vi "main.vi"() -> ()   [LabVIEW 2025]
uses:
  Controls/States.ctl
  Controls/HR_Data_Structure.ctl
  Controls/Raw_Data_IN_HR.ctl
  Controls/Runner_Data_Structure.ctl
  <vilib>/Analysis/baseanly.llb/Mean (DBL).vi
  <vilib>/Analysis/NI_AALBase.lvlib
panel:
  out "BPM":cluster{"Time":timestamp[], "Bpm":i32[]}(graph)
  out "Zone PLOT":T1(graph)
  out "Zone Data":string[][](array[string]) caption="HEART RATE ZONES"
  in  "File Path":path
  out "error out":errorcluster
  in  "error in":errorcluster
  in  "Stop":bool
  in  "Save Results":bool
  in  "New Training":bool
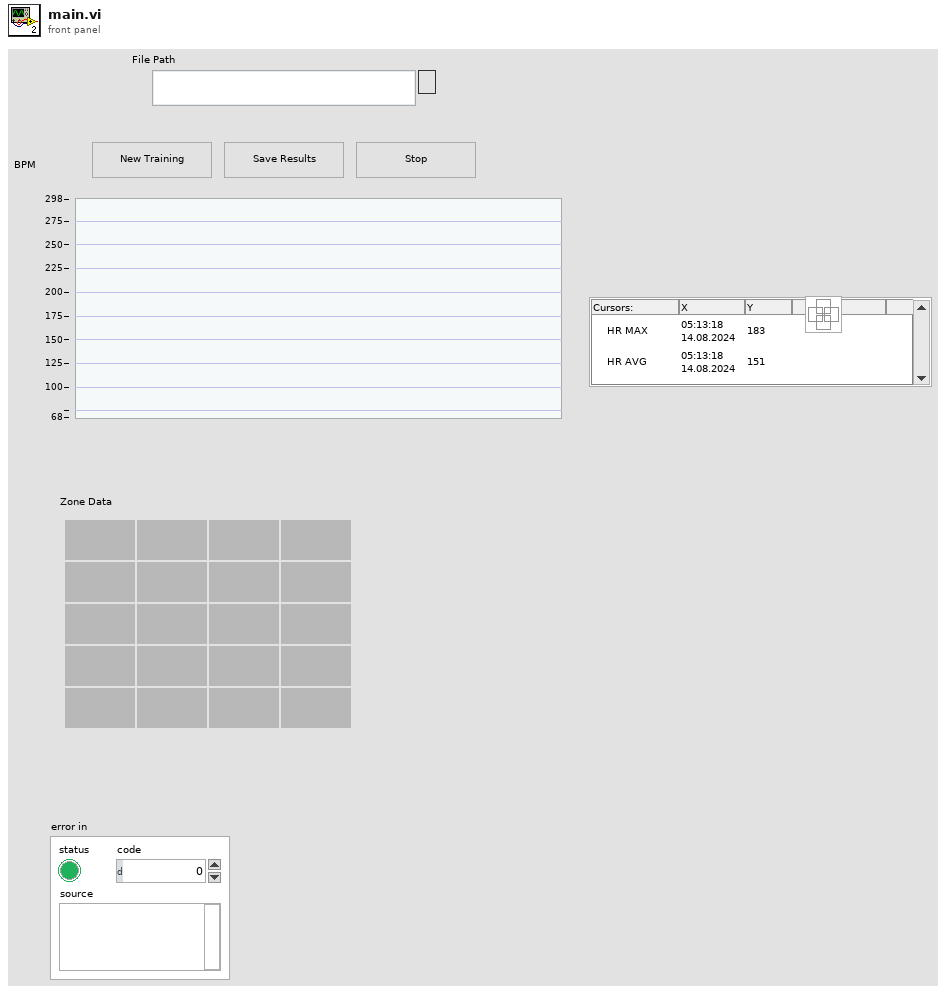
[diagram p1: front panel]
types:
  T1 = cluster{"Total Time in Zone":dbl[], "Heart Rate Zone No":dbl[]}
  T2 = typedef "HR_Data_Structure.ctl" = cluster{"HR Max":i32, "% HR MAX ":dbl[], "Raw Data":T3, "Runner's Data":T4, "HR Zone":string[][], "Total Time in Zone":dbl[], "Heart Rate Zone No":dbl[]}
  T3 = typedef "Raw_Data_IN_HR.ctl" = cluster{"Time":timestamp[], "Bpm":i32[]}
  T4 = typedef "Runner_Data_Structure.ctl" = cluster{"Name":string, "Age":i32}
  T5 = typedef "States.ctl" = enum16{"Application Error", "Init", "Idle", "Analyse New Training", "Save", "Error Handling", "Stop"}
  T6 = enum16{"open", "replace", "create", "open or create", "replace or create", "replace or create with confirmation"}
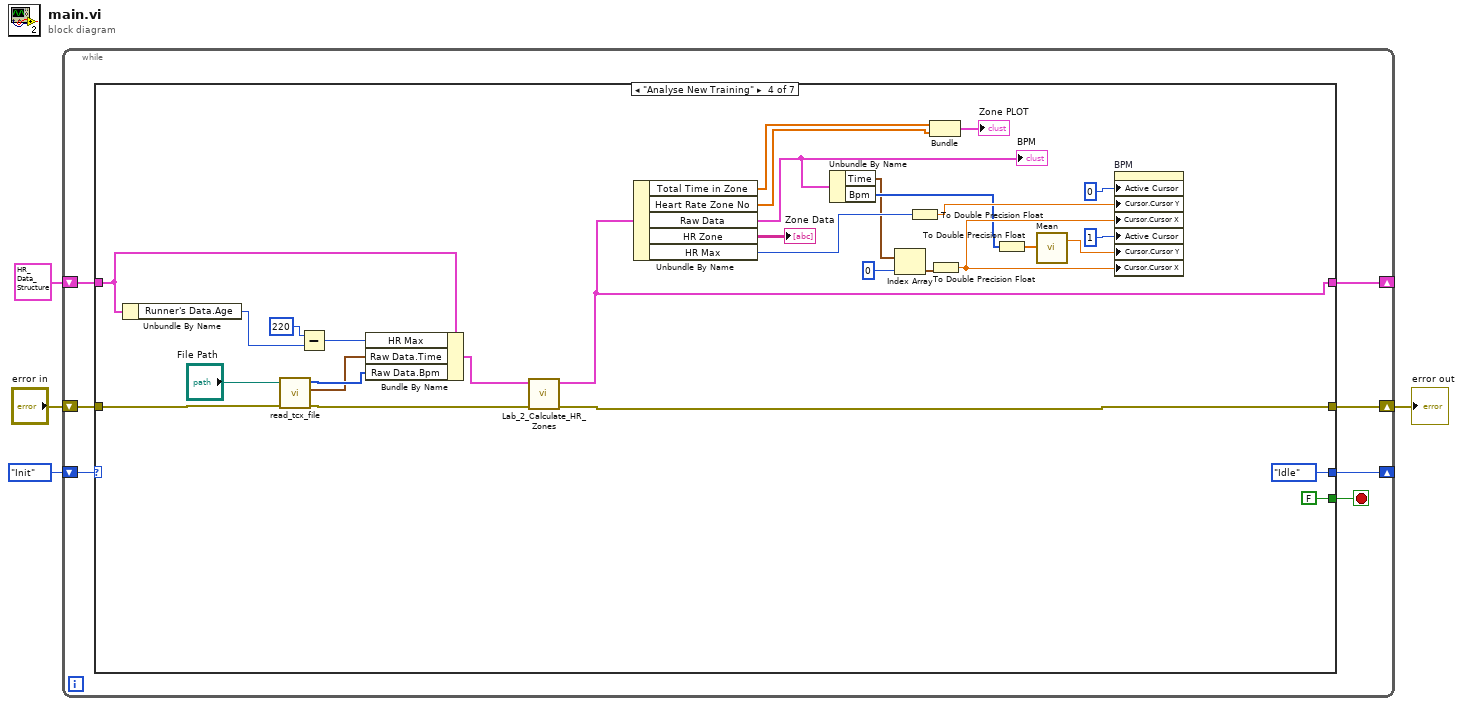
[diagram p0: block diagram]
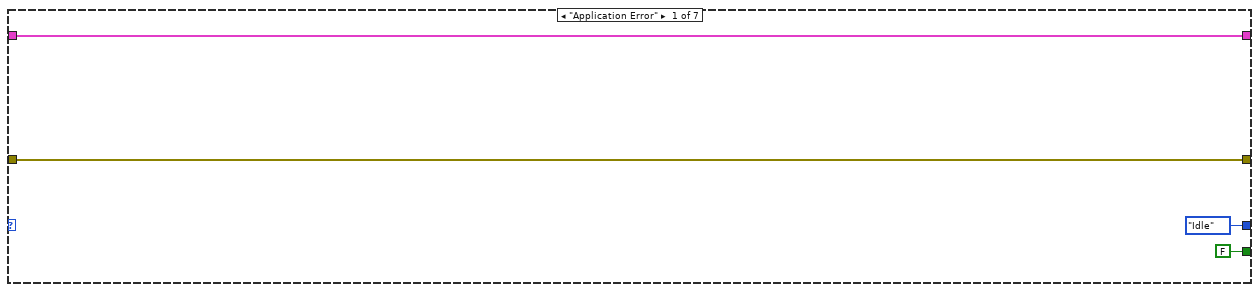
[diagram p2: hidden frame]
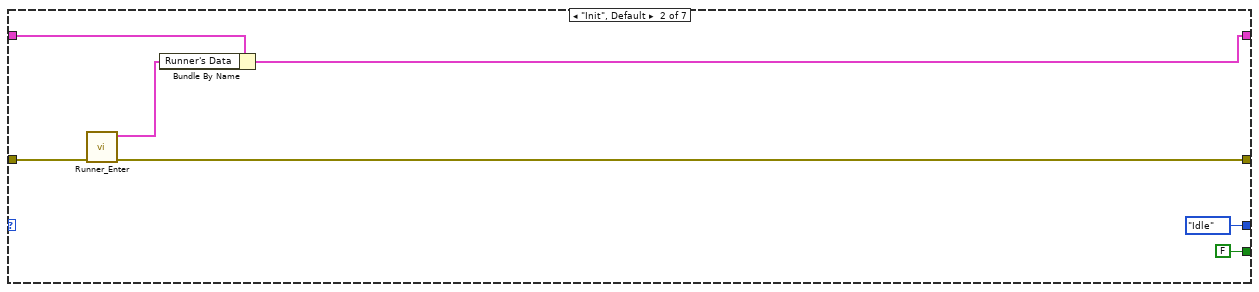
[diagram p3: hidden frame]
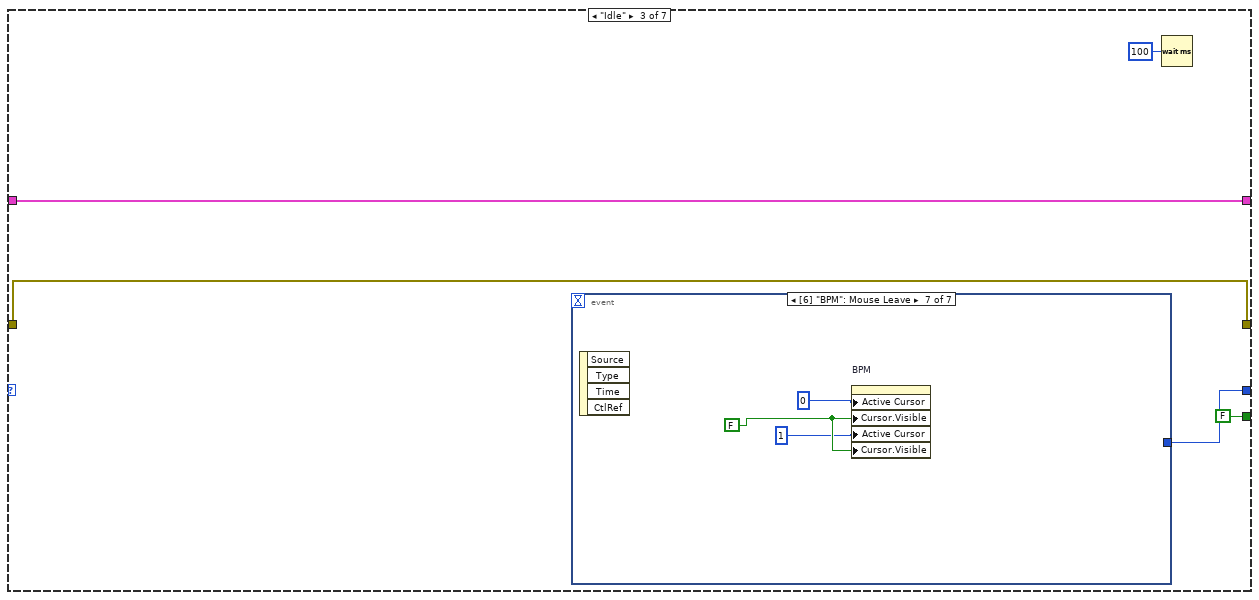
[diagram p4: hidden frame]
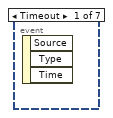
[diagram p5: hidden frame]
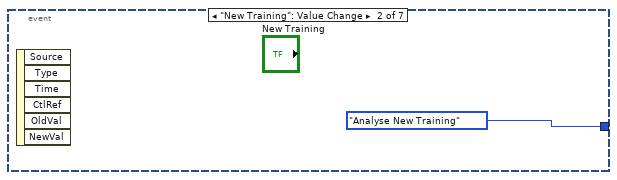
[diagram p6: hidden frame]
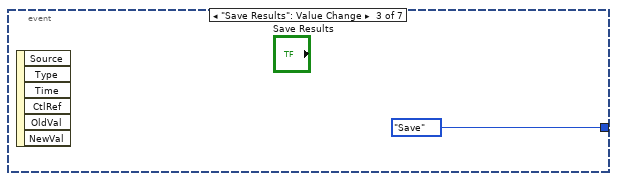
[diagram p7: hidden frame]
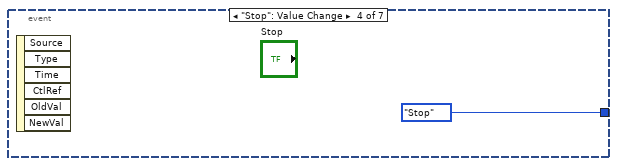
[diagram p8: hidden frame]
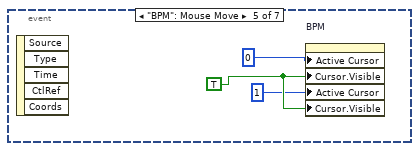
[diagram p9: hidden frame]
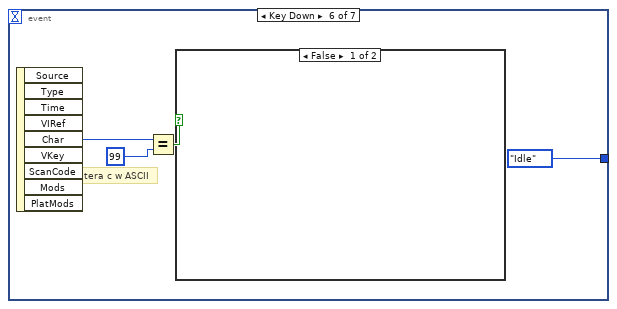
[diagram p10: hidden frame]
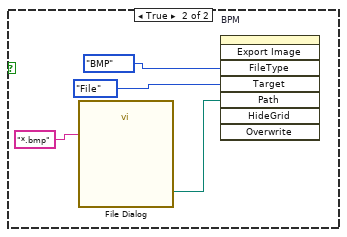
[diagram p11: hidden frame]
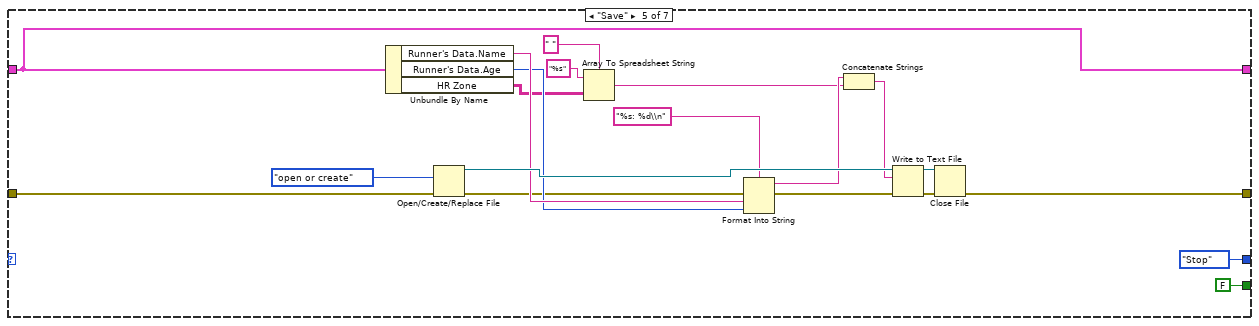
[diagram p12: hidden frame]
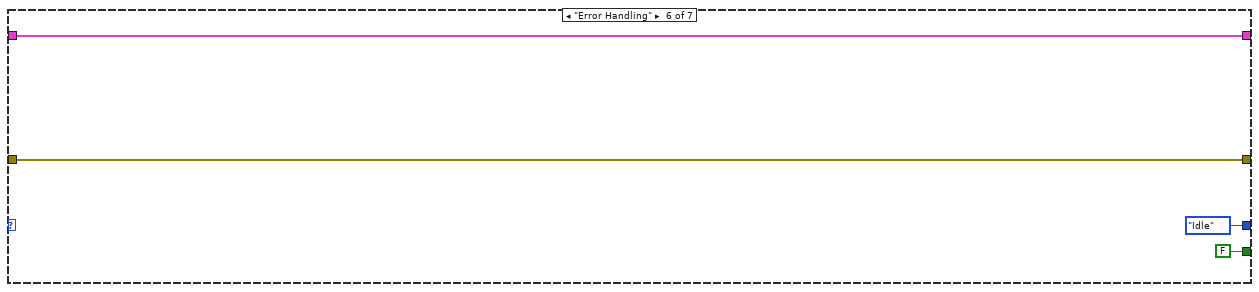
[diagram p13: hidden frame]
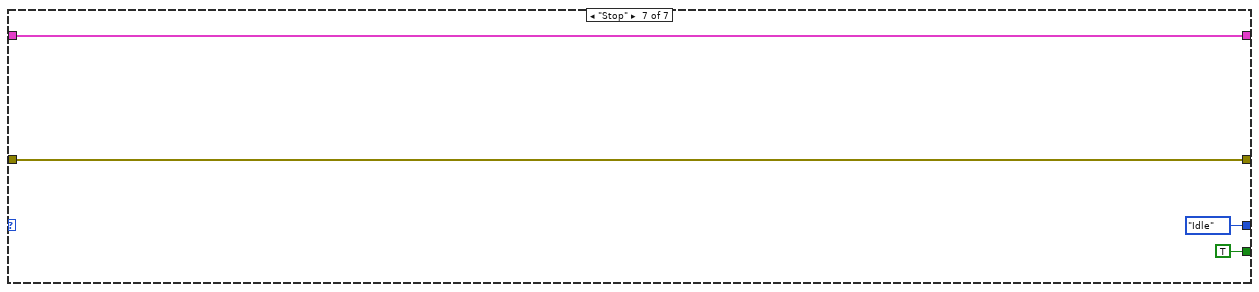
[diagram p14: hidden frame]
diagram:
  n1 = while {
    shift-right: [w11] -> _
    shift-left: States."Init" -> [w5]
    shift-right: [w8] -> _
    shift-left: T2 data[18004B] ("HR Data Structure 2") -> [w7]
    shift-right: [w9] -> w2
    shift-left: "error in" -> [w10]
    stop <- w6 stop-if-true
    n2 = case shown="\"Analyse New Training\"" w5 {
      tunnel: [States."Idle" States."Idle" w24 States."Idle" States."Stop" States."Idle" States."Idle"] -> w11
      tunnel: w10 -> [w13 w20 w27 w65 w92 w97 w101]
      tunnel: [w13 w19 w27 w74 w89 w97 w101] -> w9
      tunnel: [w14 w18 w23 w60 w88 w98 w100] -> w8
      tunnel: w7 -> [w14 w16 w23 w61 w88 w98 w100]
      tunnel: [FALSE FALSE FALSE FALSE FALSE FALSE TRUE] -> w6
      frame "Application Error" {
      }
      frame "Init", Default {
        n3 = call "Runner_Enter.vi"("error in"=w20) -> ("error out"=w19:errorcluster, "Runner's Data OUT"=w22:T4)  [unwired: 9 in]
        n4 = Bundle By Name(cluster=w16, "Runner's Data"=w22) -> (w18:T2)
      }
      frame "Idle" {
        n5 = event shown="[6] \"BPM\": Mouse Leave" {
          selector: _ -> [_ _ _ _ _ _ _]
          dyn-events: _ -> [_ _ _ _ _ _ _]
          timeout: _ -> [_ _ _ _ _ _ _]
          tunnel: [_ States."Analyse New Training" States."Save" States."Stop" _ States."Idle" _] -> w24
          event Timeout {
            n6 = event-data() -> ()  [unwired: 1 in, 3 out]
          }
          event "New Training": Value Change {
            n7 = event-data() -> ()  [unwired: 1 in, 6 out]
          }
          event "Save Results": Value Change {
            n8 = event-data() -> ()  [unwired: 1 in, 6 out]
          }
          event "Stop": Value Change {
            n9 = event-data() -> ()  [unwired: 1 in, 6 out]
          }
          event "BPM": Mouse Move {
            w33 = TRUE
            n10 = event-data() -> ()  [unwired: 1 in, 5 out]
            n11 = property on="BPM" class="XYGraph (strict)"("Active Cursor"=u32 0, "Cursor.Visible"=w33, "Active Cursor"=u32 1, "Cursor.Visible"=w33) -> ()  [unwired: 2 in, 2 out]
          }
          event Key Down {
            # "litera c w ASCII"
            n12 = event-data() -> ("Char"=w37:i16)  [unwired: 1 in, 8 out]
            n13 = Equal?(x=w37, y=i16 99) -> (x = y?=w34:bool)
            n14 = case shown="False" w34 {
              frame False {
              }
              frame True {
                n15 = call "File Dialog"("pattern (all files)"="*.bmp" ("pattern label")) -> ("selected path"=w39:path)  [unwired: 11 in, 3 out]
                n16 = invoke on="BPM" class="XYGraph (strict)" method="Export Image"("FileType"=enum32{"BMP", "EPS", "EMF", "PICT"}."BMP" ("File Type"), "Target"=enum32{"File", "Clipboard"}."File", "Path"=w39) -> ()  [unwired: 5 in, 8 out]
              }
            }
          }
          event "BPM": Mouse Leave {
            w44 = FALSE
            n17 = event-data() -> ()  [unwired: 1 in, 4 out]
            n18 = property on="BPM" class="XYGraph (strict)"("Active Cursor"=u32 0, "Cursor.Visible"=w44, "Active Cursor"=u32 1, "Cursor.Visible"=w44) -> ()  [unwired: 2 in, 2 out]
          }
        }
        n19 = Wait (ms)(milliseconds to wait=u32 100) -> ()  [unwired: 1 out]
      }
      frame "Analyse New Training" {
        n20 = Unbundle By Name(w61) -> ("Runner's Data.Age"=w73:i32)
        n21 = call "read_tcx_file.vi"("error in"=w65, "File Path"="File Path") -> ("error out"=w64:errorcluster, "Time"=w55:timestamp[], "Bmp"=w63:i32[])  [unwired: 7 in]
        n22 = Subtract(x=220, y=w73) -> (x-y=w58:i32)
        n23 = Bundle By Name(cluster=w61, "HR Max"=w58, "Raw Data.Time"=w55, "Raw Data.Bpm"=w63) -> (w71:T2)
        n24 = call "Lab_2_Calculate_HR_Zones.vi"("Error IN"=w64, "HR Data Structure IN"=w71) -> ("Error OUT"=w74:errorcluster, "HR Data Structure OUT"=w60:T2)  [unwired: 8 in]
        n25 = Unbundle By Name(w60) -> ("Total Time in Zone"=w66:dbl[], "Heart Rate Zone No"=w67:dbl[], "Raw Data"=w51:T3, "HR Zone"=→"Zone Data":string[][], "HR Max"=w50:i32)
        "BPM" <- w51
        n26 = Unbundle By Name(w51) -> ("Time"=w45:timestamp[], "Bpm"=w46:i32[])
        n27 = Index Array(array=w45, index=0) -> (element=w53:timestamp)
        n28 = To Double Precision Float(number=w50) -> (double precision float=w49:dbl)
        n29 = Bundle("Total Time in Zone"=w66, "Heart Rate Zone No"=w67) -> (→"Zone PLOT":T1)  [unwired: 1 in]
        n30 = To Double Precision Float(number=w53) -> (double precision float=w52:dbl)
        n31 = To Double Precision Float(number=w46) -> (double precision float=w48:dbl[])
        n32 = call-poly <vilib>:"Mean.vi"("X"=w48) -> ("mean"=w47:dbl)  [unwired: 1 out]
        n33 = property on="BPM" class="XYGraph (strict)"("Active Cursor"=u32 0, "Cursor.Cursor Y"=w49, "Cursor.Cursor X"=w52, "Active Cursor"=u32 1, "Cursor.Cursor Y"=w47, "Cursor.Cursor X"=w52) -> ()  [unwired: 2 in, 2 out]
      }
      frame "Save" {
        n34 = Unbundle By Name(w88) -> ("Runner's Data.Name"=w85:string, "Runner's Data.Age"=w84:i32, "HR Zone"=w81:string[][])
        n35 = Open/Create/Replace File(error in=w92, operation (0:open)=T6."open or create") -> (refnum out=w93:refnum<file>, error out=w83:errorcluster)  [unwired: 4 in, 1 out]
        n36 = Array To Spreadsheet String(delimiter (Tab)=" ", array=w81, 3:"%s" ("format string")) -> (spreadsheet string=w79:string)
        n37 = Format Into String(format string="%s: %d\\n", error in=w83, w85, w84) -> (resulting string=w80:string, error out=w82:errorcluster)  [unwired: 1 in]
        n38 = Concatenate Strings(w80, w79) -> (w78:string)
        n39 = Write to Text File(file (use dialog)=w93, text=w78, error in=w82) -> (refnum out=w91:refnum<file>, error out=w90:errorcluster)  [unwired: 1 in, 1 out]
        n40 = Close File(refnum=w91, error in=w90) -> (error out=w89:errorcluster)  [unwired: 1 out]
      }
      frame "Error Handling" {
      }
      frame "Stop" {
      }
    }
  }
  "error out" <- w2
